vi "Generator Lesson 2.vi"() -> ()   [LabVIEW 2019]
uses:
  <vilib>/Instr/_visa.llb/VISA Configure Serial Port (Instr).vi
panel:
  in  "stop":bool
  out "Waveform Chart":dbl(graph)
  in  "generator":refnum<visa-resource-name>
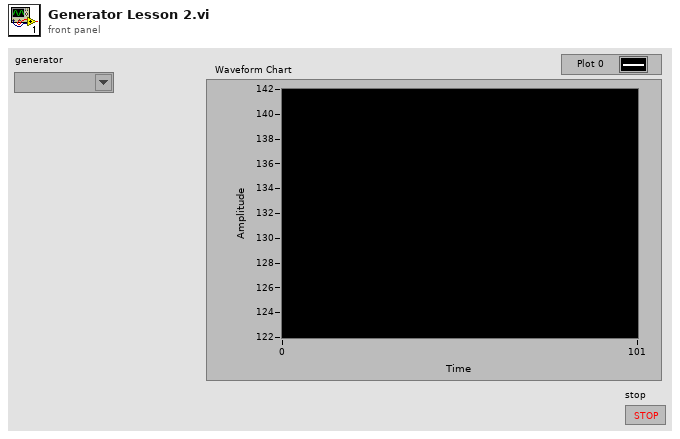
[diagram p1: front panel]
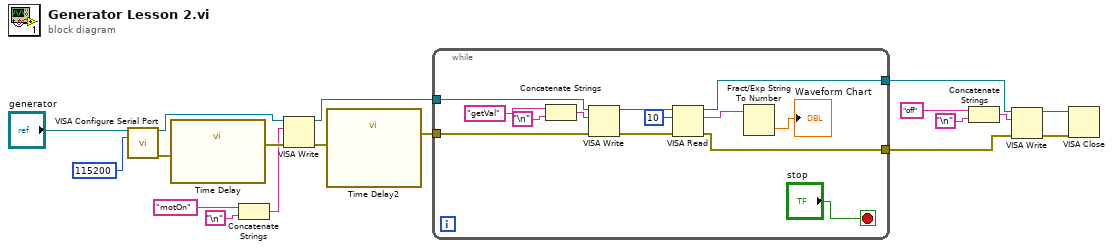
[diagram p0: block diagram]
diagram:
  n1 = call-poly "VISA Configure Serial Port"("VISA resource name"="generator", "baud rate (9600)"=u32 115200) -> ("VISA resource name out"=w15:refnum<visa-resource-name>, "error out"=w16:errorcluster)  [unwired: 12 in]
  n2 = call "Time Delay"("error in (no error)"=w16) -> ("error out"=w14:errorcluster)  [unwired: 10 in]
  n3 = Concatenate Strings("motOn", "\n") -> (w11:string)
  n4 = VISA Write(VISA resource name=w15, write buffer=w11, error in (no error)=w14) -> (VISA resource name out=w8:refnum<visa-resource-name>, error out=w10:errorcluster)  [unwired: 1 out]
  n5 = call "Time Delay2"("error in (no error)"=w10) -> ("error out"=w9:errorcluster)  [unwired: 10 in]
  n6 = while {
    tunnel: w9 -> [w29]
    tunnel: w8 -> [w28]
    tunnel: [w20] -> w4
    tunnel: [w19] -> w3
    stop <- "stop" stop-if-true
    n7 = Concatenate Strings("getVal", "\n") -> (w27:string)
    n8 = VISA Write(VISA resource name=w28, write buffer=w27, error in (no error)=w29) -> (VISA resource name out=w26:refnum<visa-resource-name>, error out=w25:errorcluster)  [unwired: 1 out]
    n9 = VISA Read(VISA resource name=w26, byte count=u32 10, error in (no error)=w25) -> (VISA resource name out=w20:refnum<visa-resource-name>, read buffer=w23:string, error out=w19:errorcluster)  [unwired: 1 out]
    n10 = Fract/Exp String To Number(string=w23) -> (number=→"Waveform Chart":dbl)  [unwired: 3 in, 1 out]
  }
  n11 = Concatenate Strings("off", "\n") -> (w5:string)
  n12 = VISA Write(VISA resource name=w4, write buffer=w5, error in (no error)=w3) -> (VISA resource name out=w2:refnum<visa-resource-name>, error out=w1:errorcluster)  [unwired: 1 out]
  n13 = VISA Close(VISA resource name=w2, error in (no error)=w1) -> ()  [unwired: 1 out]
